vi "play-AFM-raster-imaging-open-loop-singleperiod.vi"() -> ()   [LabVIEW 2017]
uses:
  <vilib>/userdefined/High Color/nirio_resource_hc.ctl
  <vilib>/Utility/file.llb/Read Delimited Spreadsheet (DBL).vi
  <vilib>/FPGAPlugInAG/cRIO-9082/niLvFpga_Open_cRIO-9082.vi
  <vilib>/rvi/interface/common/dynamic/niFpgaDynamicAddResources.vi
  <vilib>/FPGAPlugInAG/Dynamic/niLvFpga_Reset_Dynamic.vi
  <vilib>/rvi/interface/common/niFpgaWaitOnOcc.vi
  <vilib>/Utility/error.llb/Error Cluster From Error Code.vi
  <vilib>/rvi/errors/niLvFpgaAdjustHostInterfaceError.vi
  <vilib>/FPGAPlugInAG/Dynamic/niLvFpga_Run_Dynamic.vi
  <vilib>/Utility/file.llb/Write Delimited Spreadsheet (DBL).vi
  <vilib>/FPGAPlugInAG/Dynamic/niLvFpga_Close_Dynamic.vi
  <vilib>/rvi/interface/nirviOpenFPGA/nirviOpenFPGA.xnode
  FPGA Bitfiles/afmimagingcontro_FPGATargetSPARTA_raster-scanning_DXF4O8EAjZ4.lvbitx
  <vilib>/rvi/interface/nirviMethod/nirviMethod.xnode
  <vilib>/rvi/interface/nirviReadWriteControl/nirviReadWriteControl.xnode
  <vilib>/rvi/interface/nirviCloseFPGA/nirviCloseFPGA.xnode
  <vilib>/FPGAPlugInAG/Dynamic/niLvFpga_ConfigureFifo_Dynamic.vi
  <vilib>/rvi/errors/niLvFpgaMergeErrorWithErrorCode.vi
  <vilib>/rvi/interface/Simulation/niFpgaSimulationCallBeginRW.vi
  <vilib>/FPGAPlugInAG/Dynamic/niLvFpga_ReadFifo_Dynamic.vi
  NiFpgaLv.dll
  <vilib>/FPGAPlugInAG/Dynamic/niLvFpga_WriteFifo_Dynamic.vi
panel:
  out "boolean errors 2":T1
  out "Elements Remaining":u32
  in  "xy-init":fxp<+/-,16,5>[](array[numeric])=[0.0, 0.0]
  out "Actual Depth":u32
  out "size(s) 2":i32
  in  "xy-bound":sgl=7.0
  in  "reference traj path":path=path "C:/Users/arnold/Documents/labview/afm_imaging/data/data-in-singleperiod.csv"
  in  "raster-scan-params 2":T2={"TsTicks"=1600, "Stop"=FALSE, "TOL"=0.3, "ramp-rate"=-5e-05, "z-u-max"=6.0, "PI-params"={"Ki"=0.01, "setpoint"=0.5}}
  out "x+1":i32
  out "que timed out?":bool
  out "Error signal (previous line) 2":dbl[](graph)
  out "writing stopped":bool
  out "x >= y?":bool
  out "Waveform Graph":dbl[](graph)
  in  "outputData BOTH":path=path "C:/Users/arnold/Documents/labview/afm_imaging/data/data-out.csv"
  out "total_num_points":i32
  out "points_per_line":i32=250000
  out "base y_ref (ramp)":dbl[](graph)
  in  "number-of-lines":i32=256
  out "base x_ref(triangle wave)":dbl[](graph)
  out "elements left 2":i32=1
  out "(int) y*floor(x/y)":u64
  out "Empty Elements Remaining":u32
  out "nsamps 2":i32
  out "Intensity Graph":dbl[][](graph)
  in  "number-of-pixels":i32=256
  out "Error signal (previous line)":dbl[](graph)
  out "ramp-rate":sgl
  out "e(0) (threshhold init)":fxp<+/-,16,5>
  out "case-selector-feedback":i16
  in  "STOP":bool
  out "DAC-zaxis":sgl
  in  "constant 2 lower":bool
  in  "raise-constant":sgl
  out "trigger":bool
  in  "raise-constant (init)":sgl
  out "ADC-zaxis":sgl
  out "y iter":i32
  out "size(s)":i32
  in  "Ki-xy":dbl=0.005 format="%#_13g"
  # "Debug indiciators: system state"
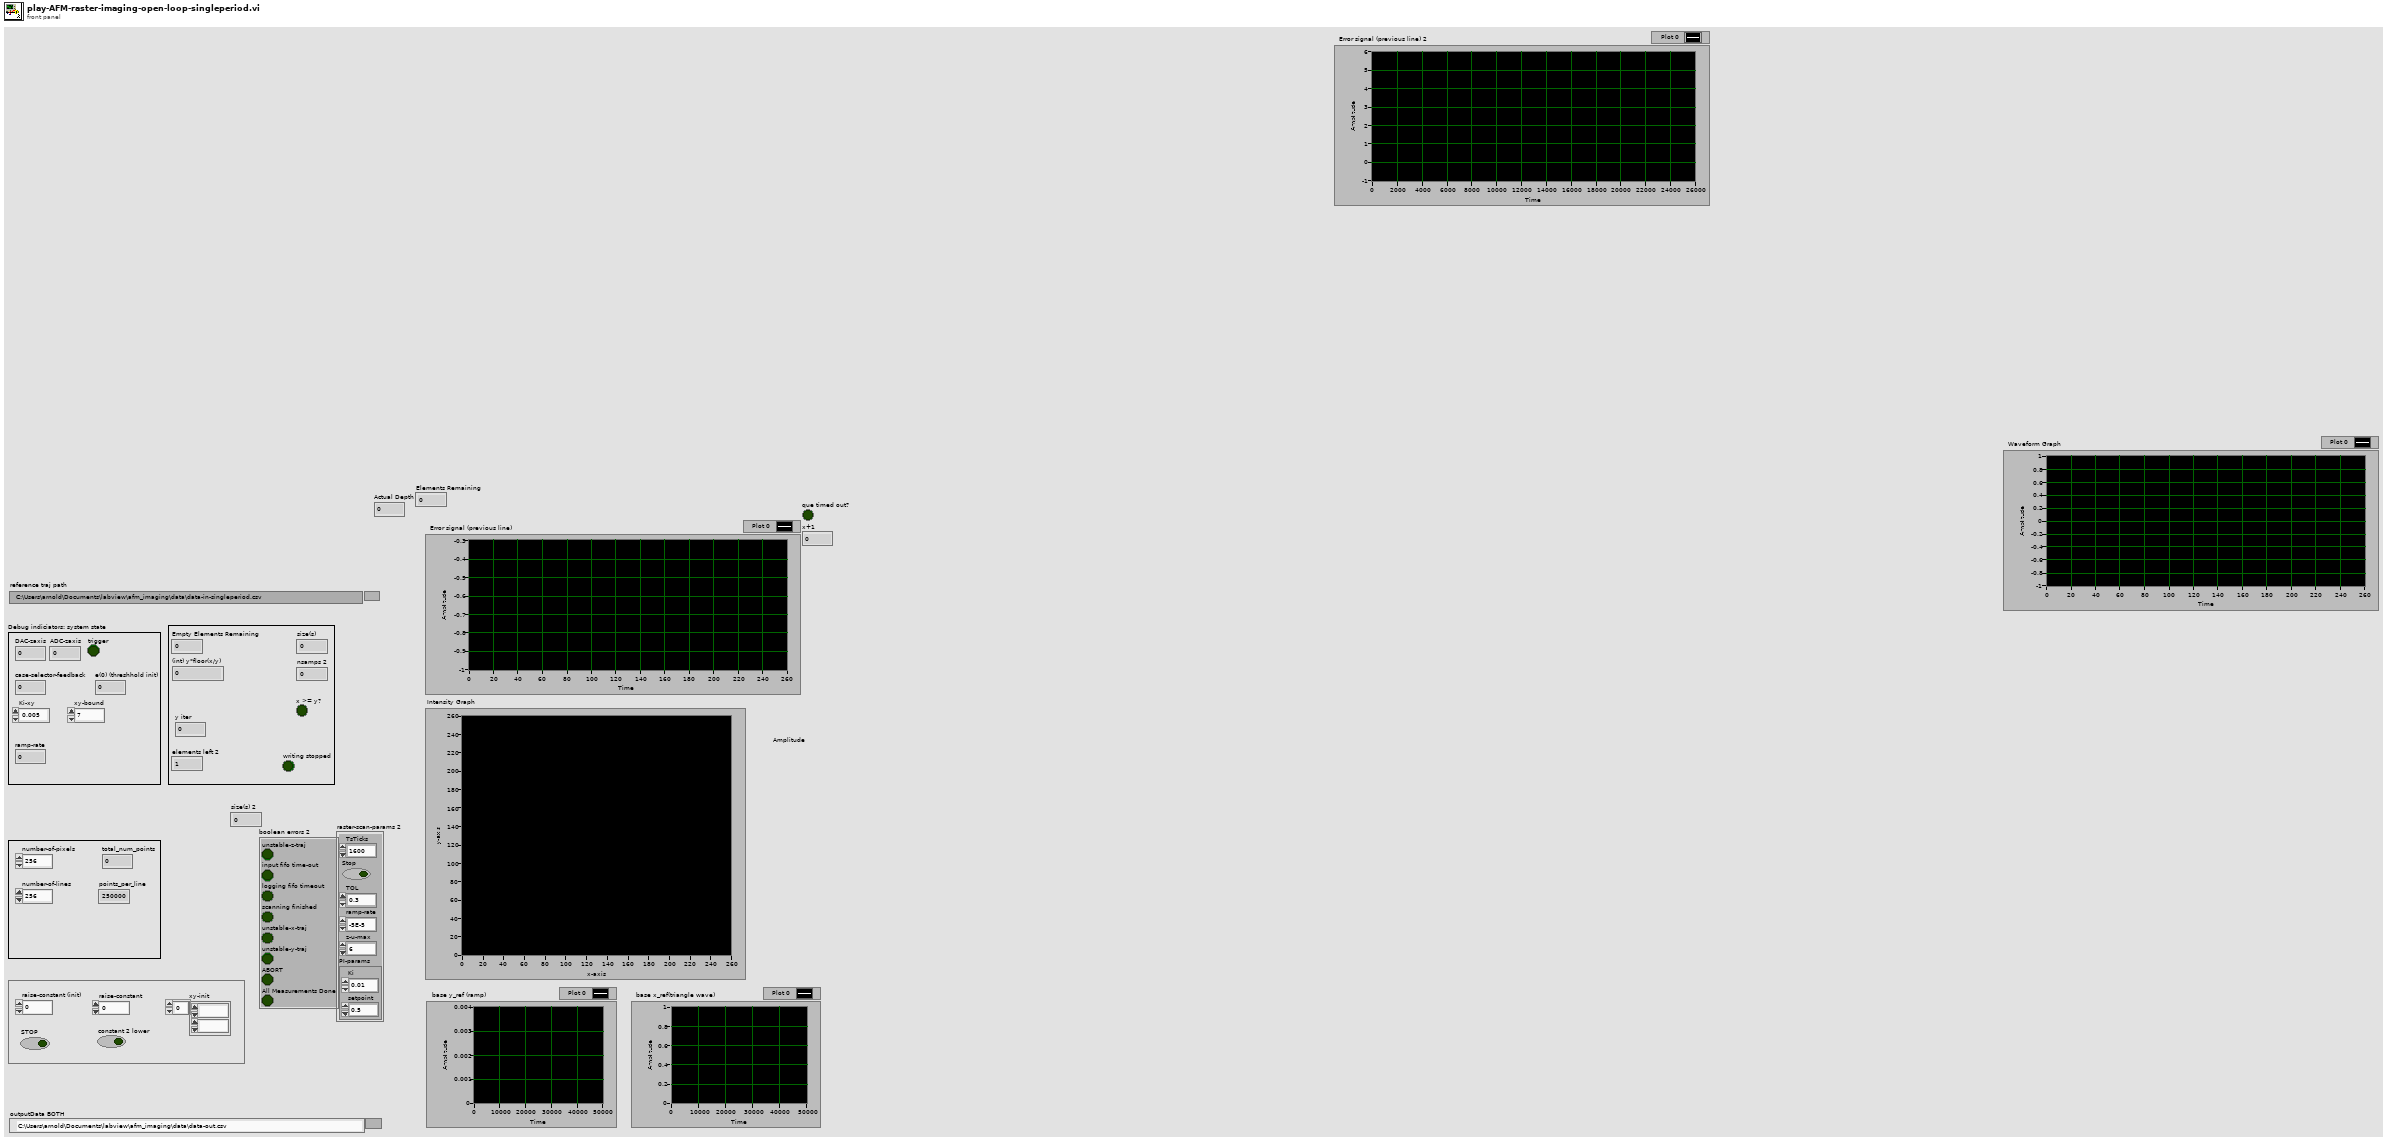
[diagram p1: front panel]
types:
  T1 = cluster{"unstable-z-traj":bool, "input fifo time-out":bool, "logging fifo timeout":bool, "scanning finished":bool, "unstable-x-traj":bool, "unstable-y-traj":bool, "ABORT":bool, "All Measurements Done":bool}
  T2 = cluster{"TsTicks":u32, "Stop":bool, "TOL":sgl, "ramp-rate":sgl, "z-u-max":sgl, "PI-params":cluster{"Ki":sgl, "setpoint":sgl}}
  T3 = typedef "nirio_resource_hc.ctl" = tag
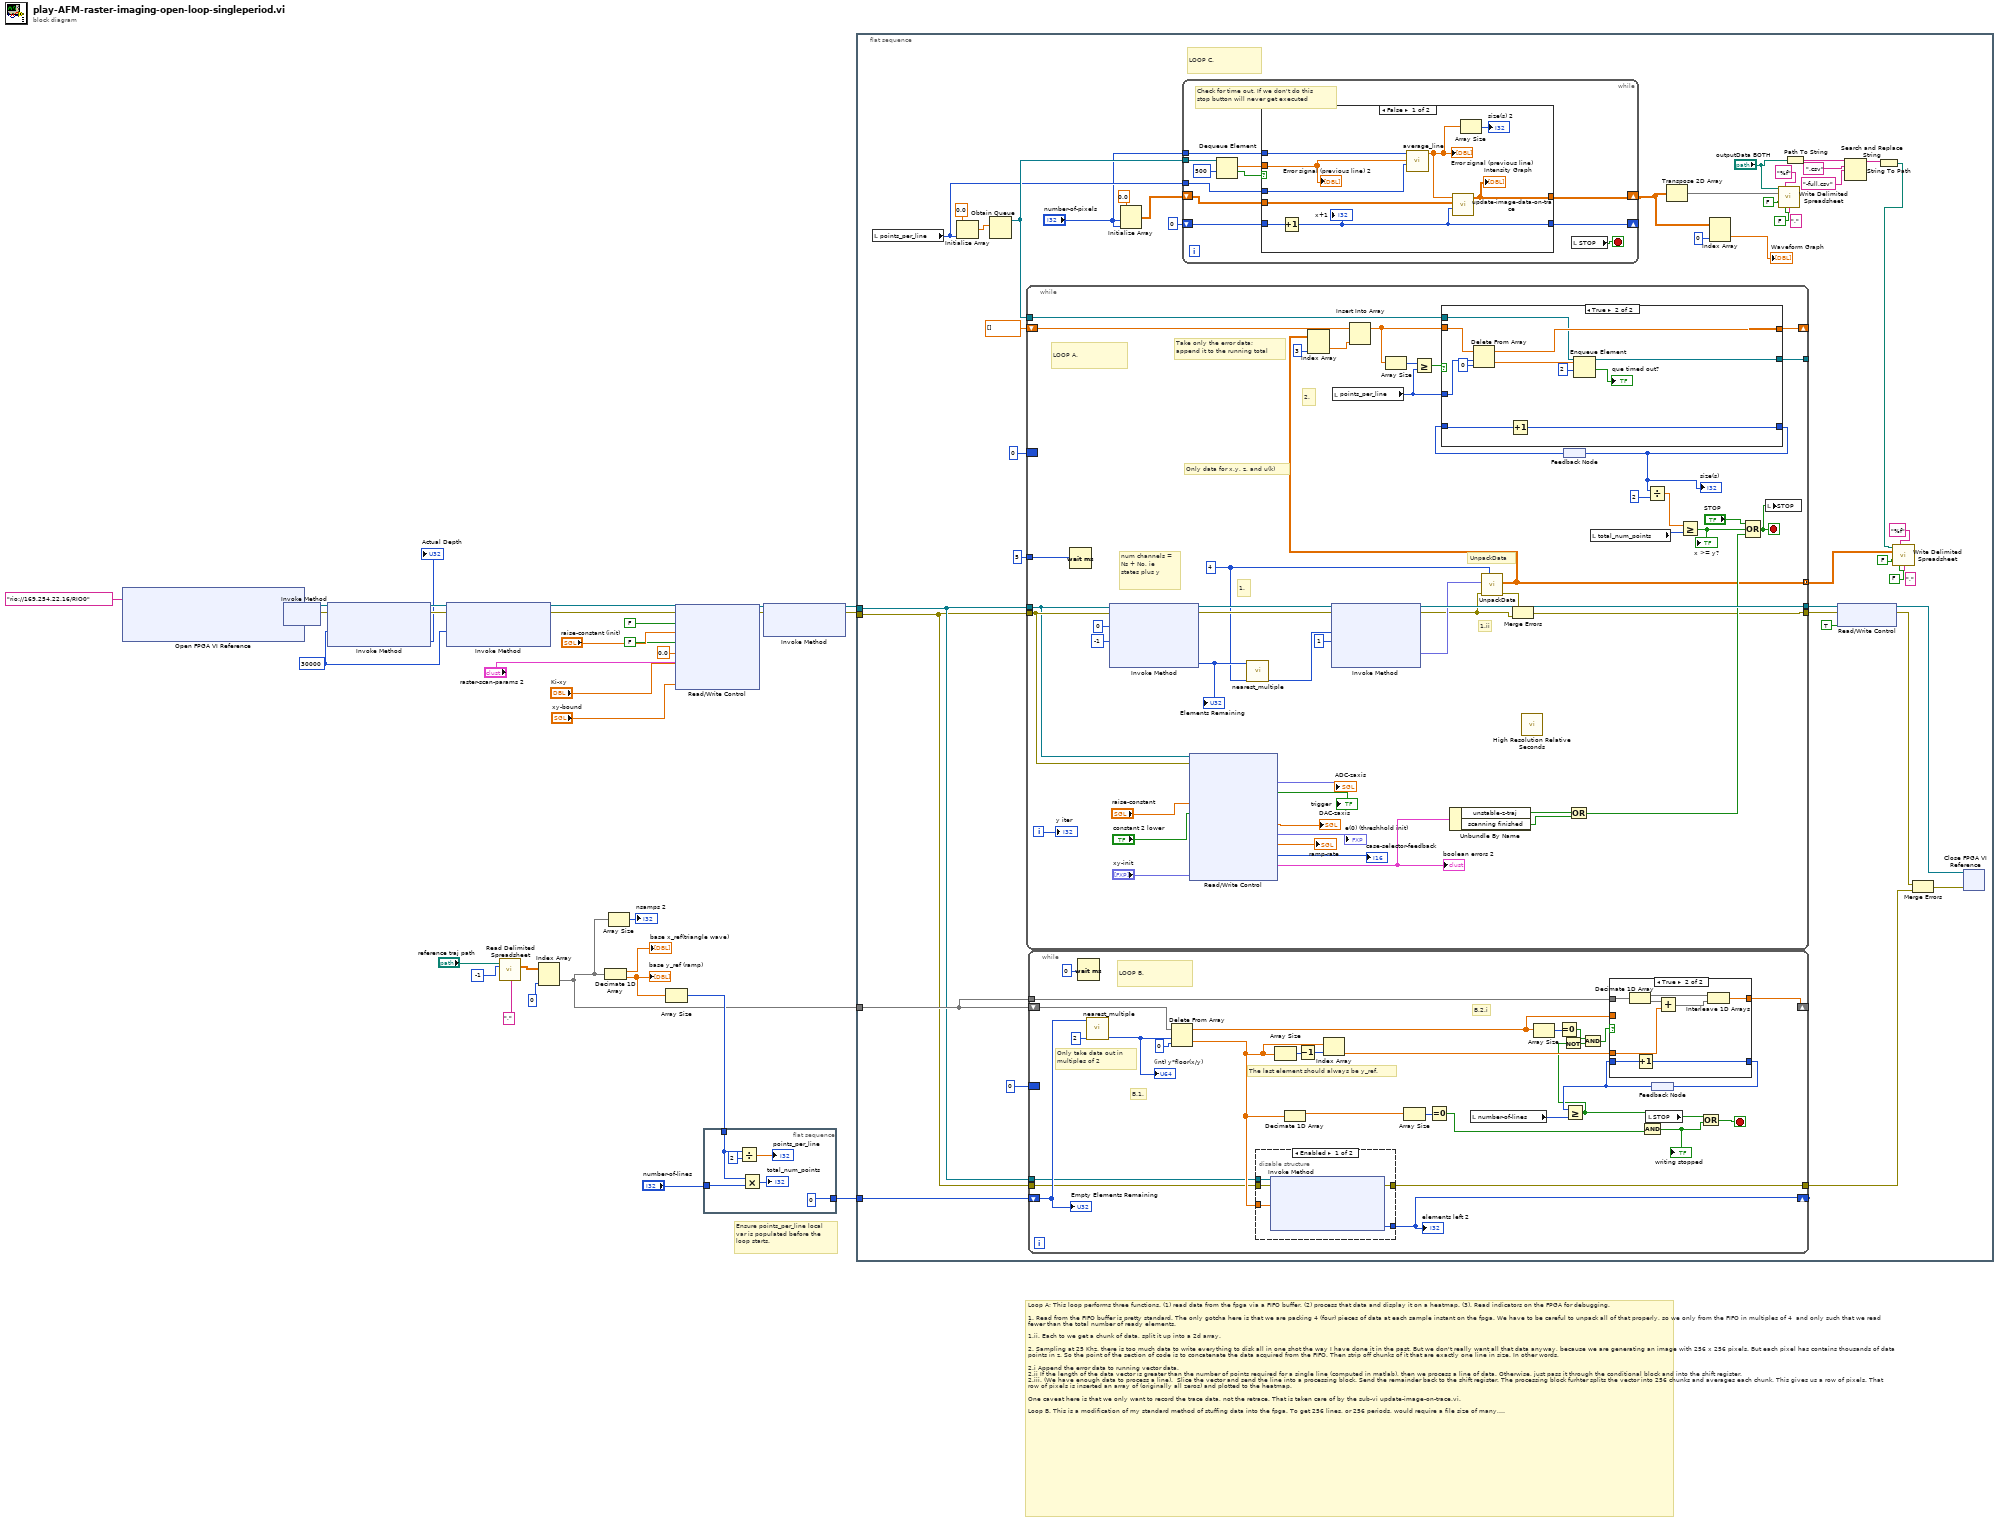
[diagram p0: block diagram]
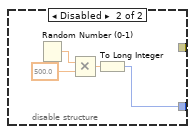
[diagram p5: hidden frame]
diagram:
  w32 = 30000
  # "Loop A; This loop performs three functions. (1) read data from the fpga via a FIFO buffer. (2) process that data and display it on a heatmap. (3). Read indicators on the FPGA for debugging.\n\n1. Read from the FIFO buffer is pretty standard. The only gotcha here is that we are packing 4 (four) pieces of data at each sample instant on the fpga. We have to be careful to unpack all of that properly, so we only from the FIFO in multiples of 4  and only such that we read fewer than the total number of ready elements. \n\n1.ii. Each to we get a chunk of data, split it up into a 2d array. \n\n2. Sampling at 25 Khz, there is too much data to write everything to disk all in one shot the way I have done it in the past. But we don't really want all that data anyway, because we are generating an image with 256 x 256 pixels. But each pixel has contains thousands of data points in z. So the point of the section of code is to concatenate the data acquired from the FIFO. Then strip off chunks of it that are exactly one line in size. In other words,\n\n2.i Append the error data to running vector data.\n2.ii If the length of the data vector is greater than the number of points required for a single line (computed in matlab), then we process a line of data. Otherwise, just pass it through the conditional block and into the shift register. \n2.iii. (We have enough data to process a line).  Slice the vector and send the line into a processing block. Send the remainder back to the shift register. The processing block furhter splits the vector into 256 chunks and averages each chunk. This gives us a row of pixels. That row of pixels is inserted an array of (originally all zeros) and plotted to the heatmap.\n\nOne caveat here is that we only want to record the trace data, not the retrace. That is taken care of by the sub-vi update-image-on-trace.vi.\n\nLoop B. This is a modification of my standard method of stuffing data into the fpga. To get 256 lines, or 256 periods, would require a file size of many, many gigibtyes. SO the point here is to only use a single period of the triangle wave and corresponding ramp signal. Everytime we exauhst that data, re-cycle the same data and keep pumping it back in. The one tricky part here is that we have to be careful to shift the original ramp data up by the appropriate amount. We also have to take special care because of how the data is packed from matlab. [x(1), y(1), x(2), y(2)...].\n\nThe first iteration of the loop, we don't push any data in. All we do is get the number of empty elements.\n\nB.1 Each iteration, strip off ' empty elements ' elements from the array and send them to FIFO. \nB.2.i Is the remaining array empty?\nB.2.ii Grab the very last element. We need this"
  # "Ensure points_per_line local\nvar is populated before the\nloop starts."
  n1 = xnode "Open FPGA VI Reference"("resource name"=T3 "rio://169.254.22.16/RIO0") -> ("FPGA VI Reference Out"=w31:refnum<k20>, "error out"=w30:errorcluster)  [unwired: 1 in]
  n2 = xnode "Invoke Method"("FPGA VI Reference In"=w31, "error in"=w30) -> ("FPGA VI Reference Out"=w26:refnum<k20>, "error out"=w25:errorcluster)
  n3 = xnode "Invoke Method"("FPGA VI Reference In"=w26, "error in"=w25, "Requested Depth"=w32) -> ("FPGA VI Reference Out"=w27:refnum<k20>, "error out"=w28:errorcluster, "Actual Depth"=→"Actual Depth":u32)
  n4 = xnode "Invoke Method"("FPGA VI Reference In"=w27, "error in"=w28, "Requested Depth"=w32) -> ("FPGA VI Reference Out"=w34:refnum<k20>, "error out"=w33:errorcluster)  [unwired: 1 out]
  n5 = call-poly <vilib>:"Read Delimited Spreadsheet.vi"("file path (dialog if empty)"="reference traj path", "number of rows (all:-1)"=-1, "delimiter (\\t)"=",") -> ("all rows"=w8:dbl[][])  [unwired: 7 in, 5 out]
  n6 = Index Array(array=w8, index (col)=0 ("dimension size")) -> (element=w7:dbl[])  [unwired: 1 in]
  n7 = Decimate 1D Array(w7) -> (→"base x_ref(triangle wave)":dbl[], w17:dbl[])
  "base y_ref (ramp)" <- w17
  n8 = Array Size(array=w7) -> (size(s)=→"nsamps 2":i32)
  n9 = Array Size(array=w17) -> (size(s)=w15:i32)
  n10 = xnode "Read/Write Control"("FPGA VI Reference In"=w34, "error in"=w33, "constant 2 lower"=FALSE, "raise-constant"="raise-constant (init)", "PID to tip up"=FALSE, "u(0)"=sgl 0.0, "raster-scan-params"="raster-scan-params 2", "Ki-xy"="Ki-xy", "xy-bound"="xy-bound") -> ("FPGA VI Reference Out"=w4:refnum<k20>, "error out"=w3:errorcluster)
  n11 = flat-sequence {
    tunnel: [0] -> w16
    tunnel: w15 -> [w36]
    tunnel: "number-of-lines" -> [w39]
    frame #0 {
      n12 = Divide(x=w36, y=2) -> (x/y=→"points_per_line":dbl)
      n13 = Multiply(x=w36, y=w39) -> (x*y=→"total_num_points":i32)
    }
  }
  n14 = xnode "Invoke Method"("FPGA VI Reference In"=w4, "error in"=w3) -> ("FPGA VI Reference Out"=w1:refnum<k20>, "error out"=w2:errorcluster)  [unwired: 1 in]
  n15 = flat-sequence {
    tunnel: w1 -> [w56]
    tunnel: w2 -> [w55]
    tunnel: w16 -> [w78]
    tunnel: w7 -> [w57]
    frame #0 {
      # "LOOP C."
      n16 = local read "points_per_line"() -> (w53:i32)
      n17 = Initialize Array(0.0 ("element"), w53) -> (w67:dbl[])
      n18 = Obtain Queue(element data type=w67) -> (queue out=w64:refnum<queue>)  [unwired: 4 in, 2 out]
      n19 = while {
        tunnel: 5 -> [w153]
        tunnel: w56 -> [w144]
        tunnel: w55 -> [w145]
        tunnel: [w121] -> w75
        tunnel: [w147] -> w77
        shift-right: [w135] -> _
        shift-left: dbl[] [] -> [w133]
        border: 0 ("disabled index (col)") -> [_]
        tunnel: w64 -> [w109]
        tunnel: [w108] -> _
        tunnel: [w106] -> w41 mode=concatenating
        i -> [w143]
        stop <- w113 stop-if-true
        w118 = u32 4 ("y")
        # "2."
        # "1.ii"
        # "1."
        # "LOOP A."
        # "Take only the error data;\nappend it to the running total"
        # "num channels = Ns + No, ie states plus y"
        # "Only data for x,y, z, and u(k)"
        # "UnpackData"
        n20 = Wait (ms)(milliseconds to wait=w153) -> ()  [unwired: 1 out]
        n21 = xnode "Invoke Method"("FPGA VI Reference In"=w144, "error in"=w145, "Number of Elements"=0 ("Timeout (ms)"), "Timeout (ms)"=-1) -> ("FPGA VI Reference Out"=w149:refnum<k20>, "error out"=w150:errorcluster, "Elements Remaining"=w119:u32)  [unwired: 1 out]
        "Elements Remaining" <- w119
        n22 = xnode "Read/Write Control"("FPGA VI Reference In"=w144, "error in"=w145, "raise-constant"="raise-constant", "constant 2 lower"="constant 2 lower", "xy-init"="xy-init") -> ("ADC-zaxis"=→"ADC-zaxis":fxp<+/-,24,5>, "trigger"=→"trigger":bool, "DAC-zaxis"=→"DAC-zaxis":sgl, "e(0) (threshhold init)"=→"e(0) (threshhold init)":fxp<+/-,16,5>, "ramp-rate"=→"ramp-rate":sgl, "current-case"=→"case-selector-feedback":i16, "boolean errors"=w105:T1)  [unwired: 1 in, 2 out]
        "boolean errors 2" <- w105
        n23 = call "nearest_multiple.vi"("numChan"=w118, "N"=w119) -> ("(int) y*floor(x/y)"=w117:u64)  [unwired: 9 in]
        n24 = xnode "Invoke Method"("FPGA VI Reference In"=w149, "error in"=w150, "Number of Elements"=w117, "Timeout (ms)"=1) -> ("FPGA VI Reference Out"=w147:refnum<k20>, "error out"=w123:errorcluster, "Data"=w146:fxp<+/-,16,5>[])  [unwired: 1 out]
        n25 = local read "points_per_line"() -> (w120:i32)
        n26 = Unbundle By Name(w105) -> ("unstable-z-traj"=w111:bool, "scanning finished"=w110:bool)
        n27 = call "UnpackData.vi"("NumChannels"=w118, "error In"=w123, "1D Data In"=w146) -> ("error Out"=w122:errorcluster, "2D Data Out"=w106:dbl[][])  [unwired: 7 in]
        n28 = Index Array(array=w106, index (col)=3 ("disabled index (col)")) -> (element=w132:dbl[])  [unwired: 1 in]
        n29 = Insert Into Array(array=w133, new element=w132) -> (w130:dbl[])  [unwired: 1 in]
        n30 = Array Size(array=w130) -> (size(s)=w134:i32)
        n31 = Greater Or Equal?(x=w134, y=w120) -> (x >= y?=w131:bool)
        n32 = Merge Errors(w122, w123) -> (w121:errorcluster)
        n33 = call <vilib>:"High Resolution Relative Seconds.vi"() -> ()  [unwired: 1 out]
        n34 = feedback #1() -> (w128:i32)
        n35 = case shown="True" w131 {
          tunnel: [w156 w165] -> w135
          tunnel: w130 -> [w156 w167]
          tunnel: w128 -> [w155 w164]
          tunnel: [w155 w163] -> w114
          tunnel: w120 -> [_ w162]
          tunnel: w109 -> [w154 w160]
          tunnel: [w154 w159] -> w108
          frame False {
          }
          frame True {
            n36 = Delete From Array(array=w167, length=w162, index=0) -> (deleted portion=w161:dbl[], array with subset deleted=w165:dbl[])
            n37 = Increment(x=w164) -> (x+1=w163:i32)
            n38 = Enqueue Element(queue=w160, element=w161, timeout in ms (-1)=2) -> (queue out=w159:refnum<queue>, timed out?=→"que timed out?":bool)  [unwired: 1 in, 1 out]
          }
        }
        "size(s)" <- w114
        n39 = feedback-in #1(w114) -> ()
        n40 = Or(x=w111, y=w110) -> (x .or. y?=w124:bool)
        n41 = local read "total_num_points"() -> (w127:i32)
        n42 = Divide(x=w114, y=2) -> (x/y=w116:dbl)
        n43 = Greater Or Equal?(x=w116, y=w127) -> (x >= y?=w125:bool)
        "x >= y?" <- w125
        n44 = Compound Arithmetic op=OR("STOP", w125, w124) -> (w113:bool)
        n45 = local write "STOP"(w113) -> ()
        "y iter" <- w143
      }
      n46 = while {
        shift-right: [w197] -> _
        shift-left: w78 -> [w192]
        shift-right: [w185] -> _
        shift-left: w57 -> [w198]
        tunnel: w57 -> [w183]
        tunnel: [w189] -> w79
        tunnel: w56 -> [w181]
        tunnel: w55 -> [w180]
        border: 0 ("Timeout (ms)") -> [_]
        stop <- w193 stop-if-true
        # "B.2.i"
        # "B.1."
        # "LOOP B."
        # "Only take data out in \nmultiples of 2"
        # "The last element should always be y_ref."
        n47 = Wait (ms)(milliseconds to wait=0) -> ()  [unwired: 1 out]
        n48 = call "nearest_multiple.vi"("numChan"=u32 2 ("Empty Elements Remaining"), "N"=w192) -> ("(int) y*floor(x/y)"=w191:u64)  [unwired: 9 in]
        "(int) y*floor(x/y)" <- w191
        n49 = Delete From Array(array=w198, length=w191, index=0) -> (deleted portion=w186:dbl[], array with subset deleted=w184:dbl[])
        n50 = disable-structure shown="Enabled" {
          disable-tunnel: [w213 w214] -> w197
          disable-tunnel: w186 -> [w212 _]
          disable-tunnel: [w211 _] -> w189
          disable-tunnel: w181 -> [w210 _]
          disable-tunnel: w180 -> [w209 _]
          frame Enabled {
            n51 = xnode "Invoke Method"("FPGA VI Reference In"=w210, "error in"=w209, "Data"=w212) -> ("error out"=w211:errorcluster, "Empty Elements Remaining"=w213:u32)  [unwired: 1 in, 1 out]
          }
          frame Disabled {
            n52 = Random Number (0-1)() -> (number: 0 to 1=w217:dbl)
            n53 = Multiply(x=w217, y=500.0) -> (x*y=w215:dbl)
            n54 = To Long Integer(number=w215) -> (32bit integer=w214:i32)
          }
        }
        "elements left 2" <- w197
        n55 = Array Size(array=w186) -> (size(s)=w187:i32)
        n56 = Decimate 1D Array(w186) -> (w172:dbl[])  [unwired: 1 out]
        n57 = Decrement(x=w187) -> (x-1=w188:i32)
        n58 = Index Array(array=w186, index=w188) -> (element=w182:dbl)
        n59 = Array Size(array=w172) -> (size(s)=w174:i32)
        n60 = Equal To 0?(x=w174) -> (x = 0?=w173:bool)
        n61 = local read "number-of-lines"() -> (w178:i32)
        n62 = Array Size(array=w184) -> (size(s)=w195:i32)
        n63 = Equal To 0?(x=w195) -> (x = 0?=w171:bool)
        n64 = local read "STOP"() -> (w194:bool)
        n65 = feedback #2() -> (w176:i32)
        n66 = Greater Or Equal?(x=w176, y=w178) -> (x >= y?=w169:bool)
        n67 = Not(x=w169) -> (.not. x?=w170:bool)
        n68 = And(x=w171, y=w170) -> (x .and. y?=w168:bool)
        n69 = case shown="True" w168 {
          tunnel: [w200 w203] -> w185
          tunnel: w184 -> [w200 _]
          tunnel: w183 -> [_ w208]
          tunnel: w182 -> [_ w206]
          tunnel: [w199 w202] -> w177
          tunnel: w176 -> [w199 w201]
          frame False {
          }
          frame True {
            n70 = Decimate 1D Array(w208) -> (w205:dbl[], w207:dbl[])
            n71 = Increment(x=w201) -> (x+1=w202:i32)
            n72 = Add(x=w207, y=w206) -> (x+y=w204:dbl[])
            n73 = Interleave 1D Arrays(w205, w204) -> (w203:dbl[])
          }
        }
        n74 = And(x=w169, y=w173) -> (x .and. y?=w175:bool)
        "writing stopped" <- w175
        n75 = feedback-in #2(w177) -> ()
        n76 = Or(x=w194, y=w175) -> (x .or. y?=w193:bool)
        "Empty Elements Remaining" <- w192
      }
      n77 = Initialize Array(0.0 ("element"), "number-of-pixels", "number-of-pixels") -> (w66:dbl[][])
      n78 = while {
        shift-right: [w93] -> w63
        shift-left: w66 -> [w92]
        shift-right: [w90] -> _
        shift-left: 0 ("disabled index (col)") -> [w91]
        tunnel: w53 -> [w89]
        tunnel: w64 -> [w88]
        tunnel: "number-of-pixels" -> [w83]
        stop <- w86 stop-if-true
        # "Check for time out. If we don't do this\nstop button will never get executed"
        n79 = Dequeue Element(queue=w88, timeout in ms (-1)=500) -> (element=w87:dbl[], timed out?=w84:bool)  [unwired: 1 in, 2 out]
        n80 = case shown="False" w84 {
          tunnel: [w102 w103] -> w93
          tunnel: w92 -> [w101 w103]
          tunnel: w91 -> [w100 w104]
          tunnel: [w99 w104] -> w90
          tunnel: w89 -> [w98 _]
          tunnel: w87 -> [w97 _]
          tunnel: w83 -> [w94 _]
          frame False {
            n81 = Increment(x=w100) -> (x+1=w99:i32)
            "x+1" <- w99
            n82 = call "average_line.vi"("data-pts-per-line"=w98, "raw-data-row"=w97, "number-of-pixels"=w94) -> ("avg-data-row"=w96:dbl[])  [unwired: 8 in]
            "Error signal (previous line)" <- w96
            n83 = call "update-image-data-on-trace.vi"("iterator"=w99, "master-image-data-n"=w101, "avg-data-row"=w96) -> ("master-image-data-out"=w102:dbl[][])  [unwired: 8 in]
            "Intensity Graph" <- w102
            n84 = Array Size(array=w96) -> (size(s)=→"size(s) 2":i32)
            "Error signal (previous line) 2" <- w97
          }
          frame True {
          }
        }
        n85 = local read "STOP"() -> (w86:bool)
      }
      n86 = Transpose 2D Array(2D array=w63) -> (transposed array=w61:dbl[][])
      n87 = Index Array(array=w63, index (col)=0 ("disabled index (col)")) -> (element=→"Waveform Graph":dbl[])  [unwired: 1 in]
      n88 = call-poly <vilib>:"Write Delimited Spreadsheet.vi"("file path (dialog if empty)"="outputData BOTH", "format (%.3f)"="%f", "2D data"=w61, "append to file? (new file:F)"=FALSE, "transpose? (no:F)"=FALSE, "delimiter (\\t)"=",") -> ()  [unwired: 8 in, 2 out]
      n89 = Path To String(path="outputData BOTH") -> (string=w46:string)
      n90 = xnode "Read/Write Control"("FPGA VI Reference In"=w77, "error in"=w75, "PID to tip up"=TRUE) -> ("FPGA VI Reference Out"=w76:refnum<k20>, "error out"=w74:errorcluster)
      n91 = Search and Replace String(input string=w46, search string=".csv" ("substring (\"\")"), replace string="-full.csv" ("substring (\"\")")) -> (result string=w43:string)  [unwired: 5 in, 3 out]
      n92 = String To Path(string=w43) -> (path=w42:path)
      n93 = call-poly <vilib>:"Write Delimited Spreadsheet.vi"("file path (dialog if empty)"=w42, "format (%.3f)"="%f", "2D data"=w41, "append to file? (new file:F)"=FALSE, "transpose? (no:F)"=FALSE, "delimiter (\\t)"=",") -> ()  [unwired: 8 in, 2 out]
      n94 = Merge Errors(w74, w79) -> (w81:errorcluster)
      n95 = xnode "Close FPGA VI Reference"("FPGA VI Reference In"=w76, "error in"=w81) -> ()  [unwired: 1 out]
    }
  }
